vi "BRD_List.vi"(10 "NewVal":T1[](array[typedef]) {"End Time" format="%<%d/%m/%Y\n%I:%M:%S %p>T"; "Start Time" format="%<%d/%m/%Y\n%I:%M:%S %p>T"}, 11 "OldVal":T1[](array[typedef]) {"End Time" format="%<%d/%m/%Y\n%I:%M:%S %p>T"; "Start Time" format="%<%d/%m/%Y\n%I:%M:%S %p>T"}) -> (1 "Boolean":bool, 2 "index of element":i32, 3 "Bootout":T1 {"End Time" format="%<%d/%m/%Y\n%I:%M:%S %p>T"; "Start Time" format="%<%d/%m/%Y\n%I:%M:%S %p>T"})   [LabVIEW 2020]
uses:
  Controls/Breakdown_List.ctl
  Controls/Loss_type.ctl
  MS SQL/MS_Global.vi
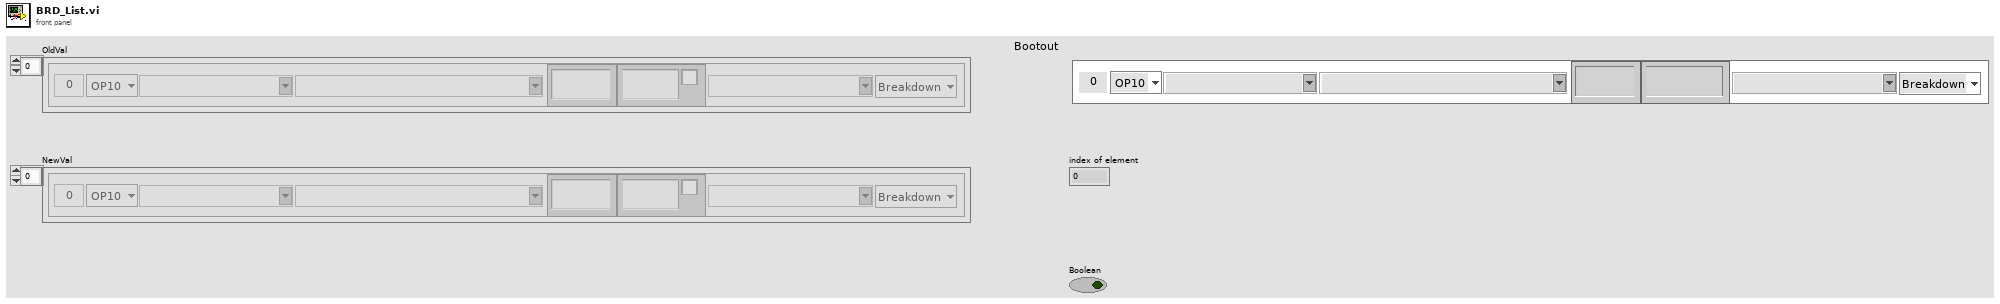
[diagram p1: front panel]
types:
  T1 = typedef "Breakdown_List.ctl" = cluster{"S.No":i32, "Reason Code":string, "Start Time":timestamp, "End Time":timestamp, "Operator":string, "Type":T2, "Machine":enum16{"OP10", "OP20", "OP30", "OP40", "OP50", "OP60", "OP70", "OP80", "LINE"}, "Reason":string}
  T2 = typedef "Loss_type.ctl" = enum16{"Breakdown", "Bookout"}
  T3 = cluster{"S.No":bool, "Reason Code":bool, "Start Time":bool, "End Time":bool, "Operator":bool, "Type":bool, "Machine":bool, "Reason":bool}[]
  T4 = cluster{"S.No":bool, "Reason Code":bool, "Start Time":bool, "End Time":bool, "Operator":bool, "Type":bool, "Machine":bool, "Reason":bool}
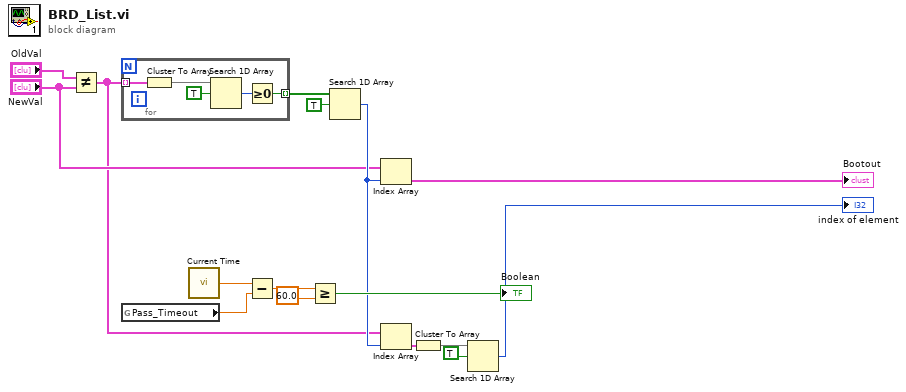
[diagram p0: block diagram]
diagram:
  n1 = Not Equal?(x="OldVal", y="NewVal") -> (x != y?=w3:T3)
  n2 = for {
    tunnel: w3 -> [w19] mode=indexing
    tunnel: [w17] -> w1 mode=indexing
    n3 = Cluster To Array(cluster=w19) -> (array=w21:bool[])
    n4 = Search 1D Array(1D array=w21, element=TRUE) -> (index of element=w18:i32)  [unwired: 1 in]
    n5 = Greater Or Equal To 0?(x=w18) -> (x >= 0?=w17:bool)
  }
  n6 = global read "MS_Global.vi" "Pass_Timeout"() -> (w11:dbl)
  n7 = call <userlib>:"Current Time.vi"() -> ("Current Time (Sec)"=w10:dbl)  [unwired: 15 in]
  n8 = Subtract(x=w10, y=w11) -> (x-y=w12:dbl)
  n9 = Greater Or Equal?(x=w12, y=60.0) -> (x >= y?=→"Boolean":bool)
  n10 = Search 1D Array(1D array=w1, element=TRUE) -> (index of element=w8:i32)  [unwired: 1 in]
  n11 = Index Array(array="NewVal", index=w8) -> (element=→"Bootout":T1)
  n12 = Index Array(array=w3, index=w8) -> (element=w4:T4)
  n13 = Cluster To Array(cluster=w4) -> (array=w5:bool[])
  n14 = Search 1D Array(1D array=w5, element=TRUE) -> (index of element=→"index of element":i32)  [unwired: 1 in]
